vi "DataProcess.vi"(10 "Data in":dbl[][](array[numeric]), 11 "element":T1) -> (0 "error out":errorcluster, 2 "Data out":dbl[][](array[numeric]))   [LabVIEW 2022 SP3]
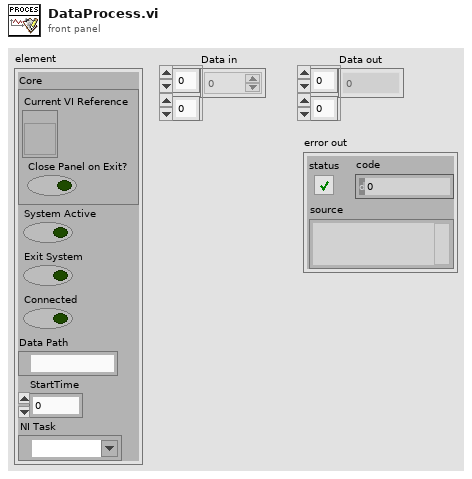
[diagram p1: front panel]
types:
  T1 = cluster{"Core":cluster{"Current VI Reference":refnum<vi>, "Close Panel on Exit?":bool}, "System Active":bool, "Exit System":bool, "Connected":bool, "Data Path":path, "StartTime":u32, "NI Task":refnum<k21>}
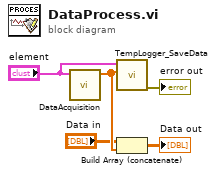
[diagram p0: block diagram]
diagram:
  n1 = call "DataAcquisition.vi"("element"="element") -> ("Data"=w5:dbl[])  [unwired: 10 in]
  n2 = call "TempLogger_SaveData.vi"("Data"=w5, "element"="element") -> ("error out"=→"error out":errorcluster)  [unwired: 9 in]
  n3 = Build Array (concatenate)("Data in", w5) -> (→"Data out":dbl[][])
